vi "SQL Execute.vi"(6 "Retries":i32, 8 "error in (no error)":errorcluster, 9 "Return Data (T)":bool=TRUE, 10 "Command Text":string, 11 "HostDB in":refnum<class "SQLite.lvclass">) -> (0 "error out":errorcluster, 1 "FirstRow":string[](array[string]), 2 "Table Control":string[][](table), 3 "HostDB out":refnum<class "SQLite.lvclass">, 4 "Rows Fetched":i32)   [LabVIEW 2021, in "SQLite.lvclass"]
uses:
  SQLite.lvclass
  <vilib>/drjdpowell/SQLite Library/SQL Connection/Execute SQL (No results).vi
  <vilib>/drjdpowell/SQLite Library/SQL Connection/Connection.lvclass
  <userlib>/sushu/sushu.lvlib
  <vilib>/drjdpowell/SQLite Library/SQLite.lvlib
panel:
  # "----------------------------------------\n2021-07-09 16:04:01.401\nCall Chain:\nSQLite.lvclass:SQL Execute.vi\n\nUserMessage: \n--------------------\nINSERT INTO OP140_3\n(\nItemsID,MainBarcode,ProductNum,StartDate,Result,ResultsNum\n)\n VALUES \n(\n'0','Idle_2021-07-03-214821','JQM-11C','2021-07-03 21:48:21','NG','17','2021-07-03 21:48:21','0','Idle_2021-07-03-214821','OP140_3','0','0','JQM-11C','0','0','0','0','2021-07-03 21:48:21','Auto','D:\\ResultsData\\2021-07-03\\OP140_3\\JQM-11C\\Idle-2021-07-03-214821_Idle.tdms','0','NG','0.000'\n)\nCall Chain: \nSQLite.lvclass:SQL Execute.vi\n--------------------\n\n----------------------------------------"
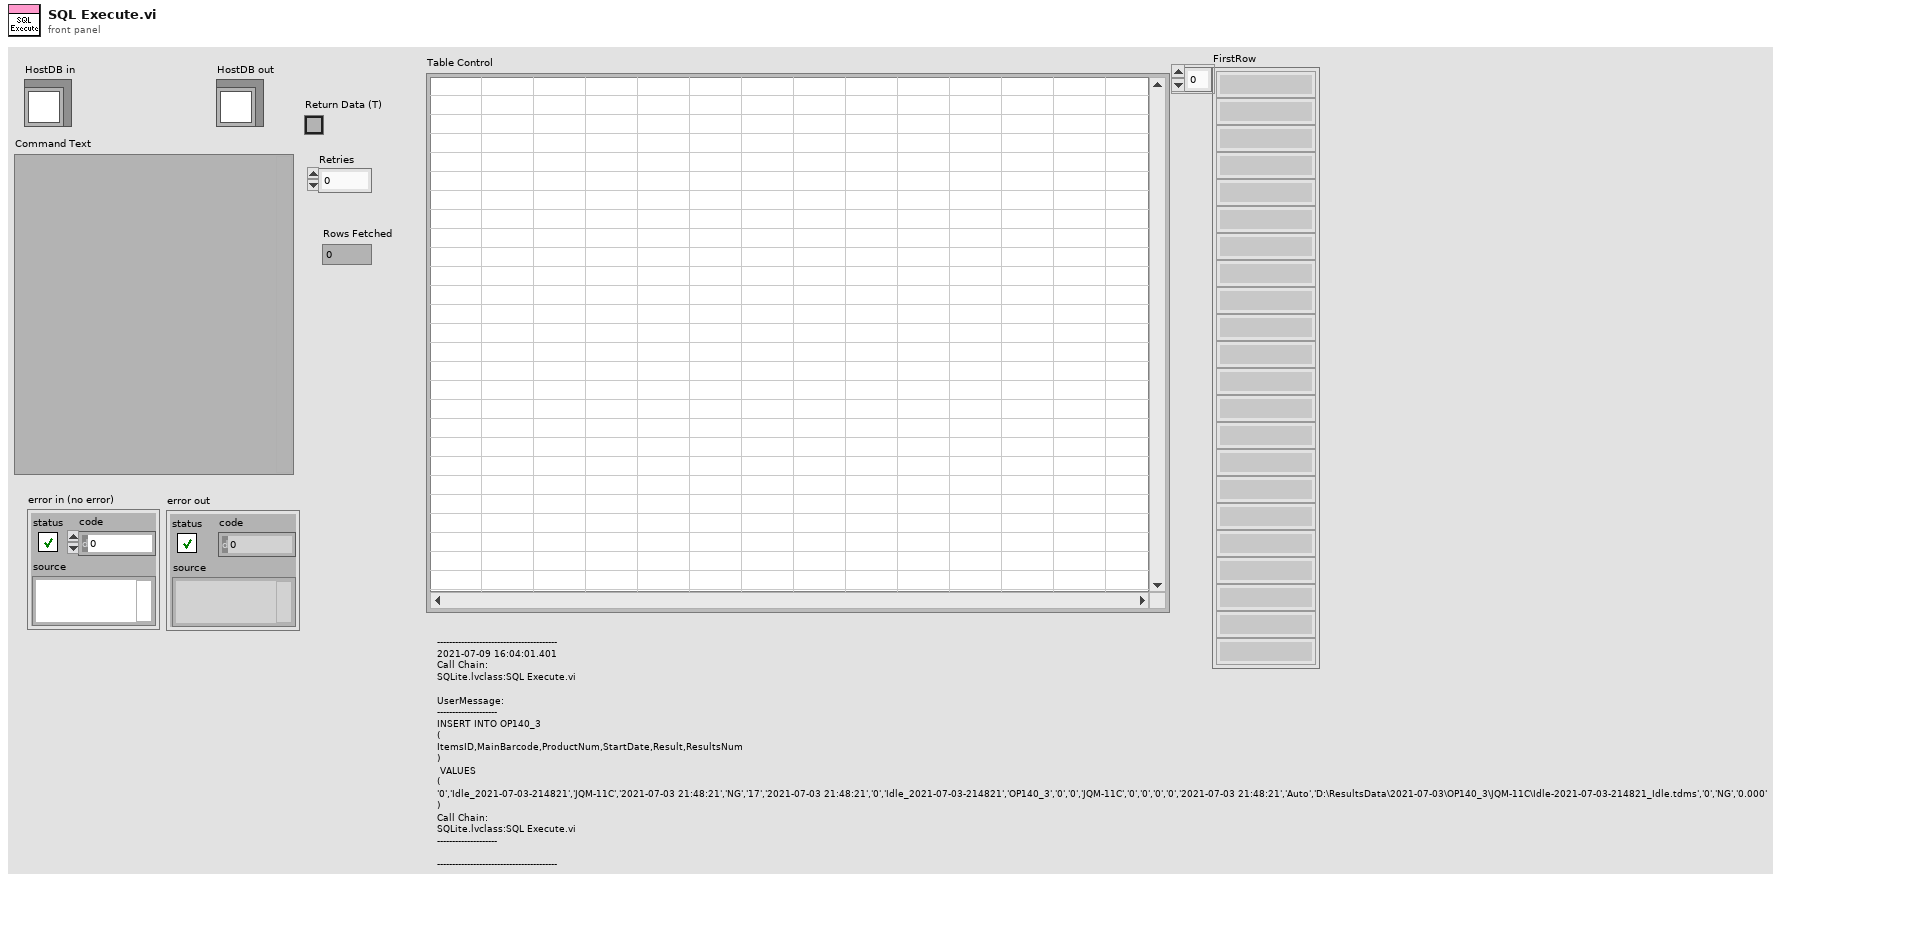
[diagram p1: front panel]
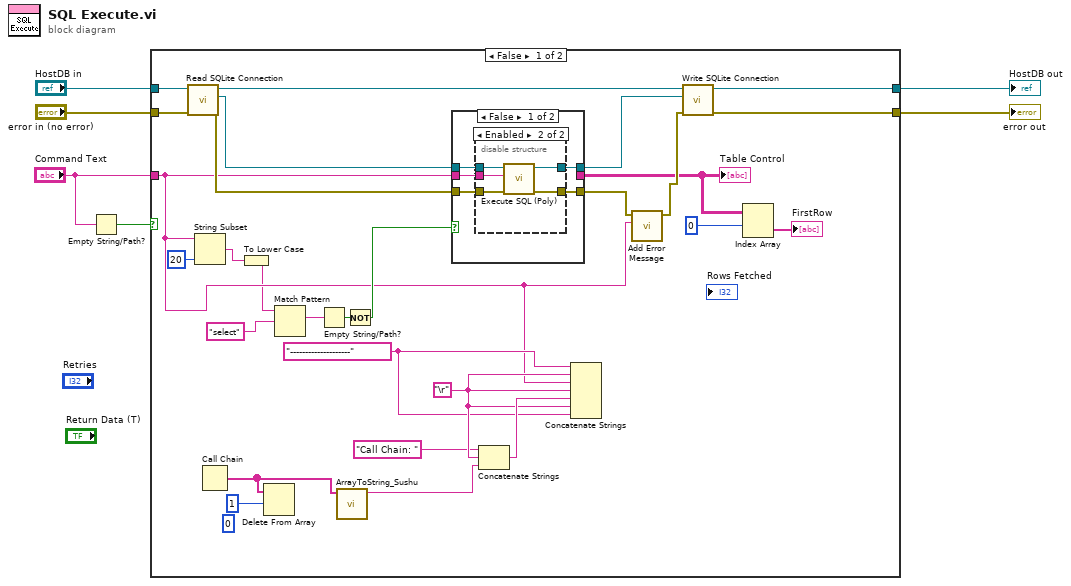
[diagram p0: block diagram]
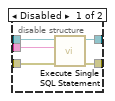
[diagram p2: hidden frame]
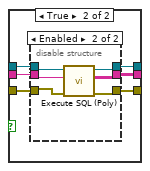
[diagram p3: hidden frame]
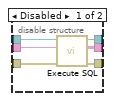
[diagram p4: hidden frame]
diagram:
  n1 = Empty String/Path?(string/path="Command Text") -> (empty?=w1:bool)
  n2 = case shown="False" w1 {
    tunnel: "HostDB in" -> [w34 w69]
    tunnel: [w30 w69] -> w5
    tunnel: "error in (no error)" -> [w29 w68]
    tunnel: [w27 w68] -> w3
    tunnel: "Command Text" -> [w10 _]
    frame False {
      (unwired) 0 ("index")
      w11 = "--------------------" ("string")
      w15 = "\r"
      n3 = call-dynamic "Read SQLite Connection.vi"("error in (no error)"=w29, "SQLite in"=w34) -> ("error out"=w28:errorcluster, "SQLite.lvlib:Connection"=w33:refnum<class "Connection.lvclass">, "SQLite out"=w32:refnum<class "SQLite.lvclass">)  [unwired: 7 in]
      n4 = String Subset(string=w10, length (rest)=20 ("length (rest)")) -> (substring=w8:string)  [unwired: 1 in]
      n5 = Call Chain() -> (call chain=w13:string[])
      n6 = To Lower Case(string=w8) -> (all lower case string=w7:string)
      n7 = Delete From Array(array=w13, length=1) -> ()  [unwired: 1 in, 2 out]
      n8 = Match Pattern(string=w7, regular expression="select") -> (match substring=w23:string)  [unwired: 1 in, 3 out]
      n9 = Empty String/Path?(string/path=w23) -> (empty?=w24:bool)
      n10 = call <userlib>:"ArrayToString_Sushu.vi"("Array"=w13) -> ("String"=w16:string)  [unwired: 10 in]
      n11 = Not(x=w24) -> (.not. x?=w21:bool)
      n12 = case shown="False" w21 {
        tunnel: w33 -> [w39 w55]
        tunnel: [_ w54] -> w18
        tunnel: [w38 w53] -> w31
        tunnel: w28 -> [w36 w52]
        tunnel: [w35 w51] -> w25
        tunnel: w10 -> [w37 w50]
        frame False {
          n13 = disable-structure shown="Enabled" {
            disable-tunnel: w39 -> [w44 w49]
            disable-tunnel: [w43 w47] -> w38
            disable-tunnel: w37 -> [w42 w48]
            disable-tunnel: w36 -> [w41 w46]
            disable-tunnel: [w40 w45] -> w35
            frame Disabled {
              n14 = call <vilib>:"Execute Single SQL Statement.vi"("error in (no error)"=w41, "SQL statement"=w42, "SQLite Connection in"=w44) -> ("error out"=w40:errorcluster, "SQLite Connection"=w43:refnum<class "Connection.lvclass">)  [unwired: 7 in]
            }
            frame Enabled {
              n15 = call-poly <vilib>:"Execute SQL (Poly).vi"("error in (no error)"=w46, "SQL"=w48, "SQLite Connection in"=w49) -> ("error out"=w45:errorcluster, "SQLite Connection"=w47:refnum<class "Connection.lvclass">)  [unwired: 7 in]
            }
          }
        }
        frame True {
          n16 = disable-structure shown="Enabled" {
            disable-tunnel: w55 -> [w61 w67]
            disable-tunnel: [w60 w62] -> w54
            disable-tunnel: [w59 w66] -> w53
            disable-tunnel: w52 -> [w58 w65]
            disable-tunnel: [w57 w63] -> w51
            disable-tunnel: w50 -> [w56 w64]
            frame Disabled {
              n17 = call <vilib>:"Execute SQL.vi"("error in (no error)"=w58, "SQL"=w56, "SQLite Connection in"=w61) -> ("error out"=w57:errorcluster, "Result Set"=w60:string[][], "SQLite Connection"=w59:refnum<class "Connection.lvclass">)  [unwired: 5 in, 1 out]
            }
            frame Enabled {
              n18 = call-poly <vilib>:"Execute SQL (Poly).vi"("error in (no error)"=w65, "SQL"=w64, "SQLite Connection in"=w67) -> ("error out"=w63:errorcluster, "Result Set"=w62:string[][], "SQLite Connection"=w66:refnum<class "Connection.lvclass">)  [unwired: 5 in, 1 out]
            }
          }
        }
      }
      "Table Control" <- w18
      n19 = Concatenate Strings("Call Chain: " ("string"), w15, w16) -> (w17:string)
      n20 = Concatenate Strings(w11, w15, w10, w15, w17, w15, w11) -> ()  [unwired: 1 out]
      n21 = call <userlib>:"Add Error Message.vi"("ErrorMessages"=w10, "error in (no error)"=w25) -> ("error out"=w26:errorcluster)  [unwired: 9 in]
      n22 = call-dynamic "Write SQLite Connection.vi"("error in (no error)"=w26, "SQLite.lvlib:Connection"=w31, "SQLite in"=w32) -> ("error out"=w27:errorcluster, "SQLite out"=w30:refnum<class "SQLite.lvclass">)  [unwired: 7 in]
      n23 = Index Array(array=w18, index (row)=0) -> (element=→"FirstRow":string[])  [unwired: 1 in]
    }
    frame True {
    }
  }
  "error out" <- w3
  "HostDB out" <- w5
